vi "Boolean Functional Global.vi"(10 "Input Bool":bool, 11 "Action":enum16{"Set Data", "Get Data"}(ring)) -> (3 "Output Bool":bool)   [LabVIEW 2014]
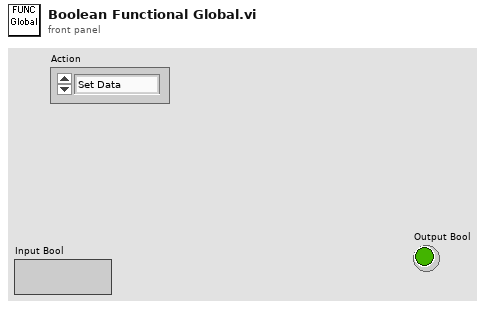
[diagram p1: front panel]
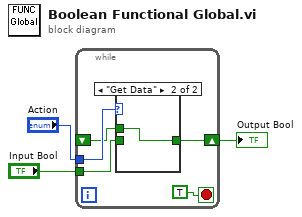
[diagram p0: block diagram]
diagram:
  n1 = while {
    shift-right: [w6] -> w2
    shift-left: _ -> [w7]
    tunnel: "Action" -> [w8]
    tunnel: "Input Bool" -> [w5]
    stop <- TRUE stop-if-true
    n2 = case shown="\"Get Data\"" w8 {
      tunnel: w7 -> [_ w10]
      tunnel: [w9 w10] -> w6
      tunnel: w5 -> [w9 _]
      frame "Set Data", Default {
      }
      frame "Get Data" {
      }
    }
  }
  "Output Bool" <- w2
